vi "VI Server_CtlRef_Generic_Get.vi"(7 "Control.Label":string, 8 "error in":errorcluster, 9 "SingleInstance":bool, 11 "VI Server.RefsCluster":T1) -> (0 "error out":errorcluster, 1 "Control.Ref.Generic":refnum<vi>, 3 "VI Server.RefsCluster.DUP":T1)   [LabVIEW 2020]
uses:
  VI Server_TypeDefs/VI Server_RefsCluster.ctl
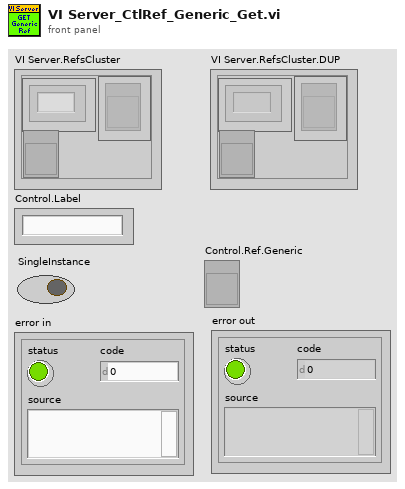
[diagram p1: front panel]
types:
  T1 = typedef "VI Server_RefsCluster.ctl" = cluster{"Labels":string[], "Refs":refnum<vi>[], "VI Ref":refnum<vi>}
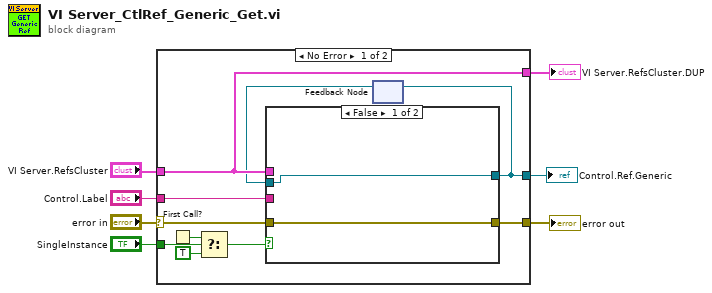
[diagram p0: block diagram]
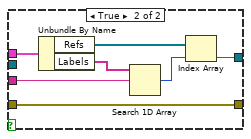
[diagram p2: hidden frame]
diagram:
  n1 = case shown="No Error" "error in" {
    selector: "error in" -> [w16 w27]
    tunnel: "VI Server.RefsCluster" -> [w15 _]
    tunnel: "Control.Label" -> [w17 _]
    tunnel: [w8 w27] -> w4
    tunnel: [w9 _] -> w1
    tunnel: [w15 _] -> w3
    tunnel: "SingleInstance" -> [w14 _]
    frame No Error {
      n2 = First Call?() -> (First Call?: T/F=w12:bool)
      n3 = Select(t=w12, s=w14, f=TRUE) -> (s? t:f=w13:bool)
      n4 = feedback #1() -> (w10:refnum<vi>)  [unwired: 1 in]
      n5 = case shown="False" w13 {
        tunnel: w17 -> [_ w25]
        tunnel: w16 -> [w18 w21]
        tunnel: [w18 w21] -> w8
        tunnel: [w19 w22] -> w9
        tunnel: w15 -> [_ w20]
        tunnel: w10 -> [w19 _]
        frame False {
        }
        frame True {
          n6 = Unbundle By Name(w20) -> ("Refs"=w24:refnum<vi>[], "Labels"=w26:string[])
          n7 = Search 1D Array(1D array=w26, element=w25) -> (index of element=w23:i32)  [unwired: 1 in]
          n8 = Index Array(array=w24, index=w23) -> (element=w22:refnum<vi>)
        }
      }
      n9 = feedback-in #1(w9) -> ()
    }
    frame Error {
    }
  }
  "VI Server.RefsCluster.DUP" <- w3
  "error out" <- w4
  "Control.Ref.Generic" <- w1
